vi "test.vi"() -> ()   [LabVIEW 2021]
uses:
  <vilib>/gmath/NI_Gmath.lvlib
panel:
  in  "formula":string
  out "y value":dbl format="%.2f"
  out "element":string
  out "error out":errorcluster
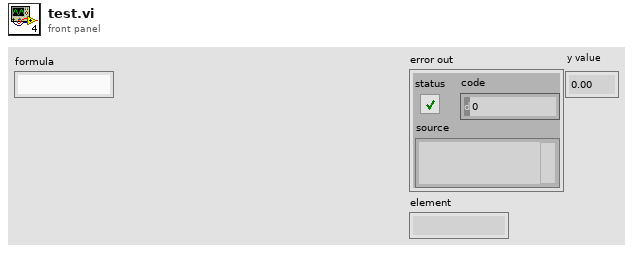
[diagram p1: front panel]
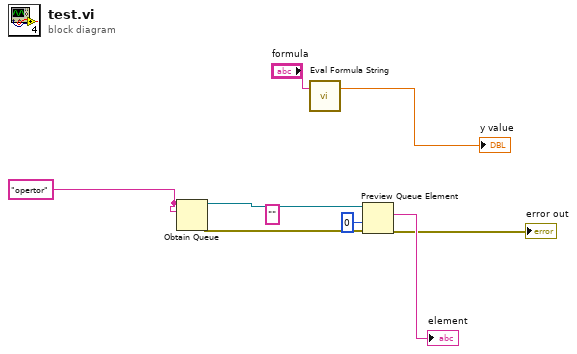
[diagram p0: block diagram]
diagram:
  (unwired) "" ("element")
  w8 = "opertor" ("name (unnamed)")
  n1 = Obtain Queue(name (unnamed)=w8, element data type=w8) -> (queue out=w6:refnum<queue>, error out=w5:errorcluster)  [unwired: 3 in, 1 out]
  n2 = call <vilib>:"Eval Formula String.vi"("formula"="formula") -> ("y value"=→"y value":dbl)  [unwired: 1 in, 1 out]
  n3 = Preview Queue Element(queue=w6, timeout in ms (-1)=0, error in (no error)=w5) -> (element=→"element":string, error out=→"error out":errorcluster)  [unwired: 2 out]
